vi "COM Error Checker.vi"(2 "error in (no error)":errorcluster, 3 "String In":string) -> (0 "error out":errorcluster, 1 "String":string)   [LabVIEW 2019, in "Instrument.KH7008.lvclass"]
uses:
  Instrument.KH7008.lvclass
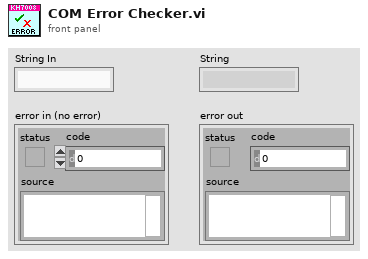
[diagram p1: front panel]
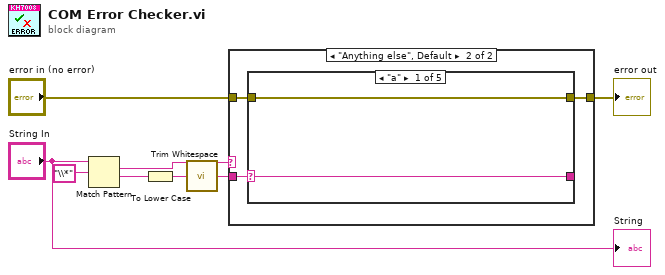
[diagram p0: block diagram]
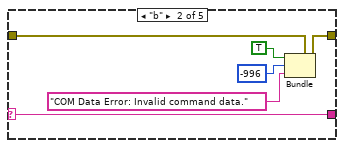
[diagram p3: hidden frame]
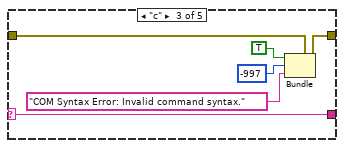
[diagram p4: hidden frame]
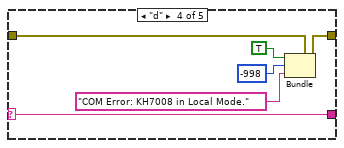
[diagram p5: hidden frame]
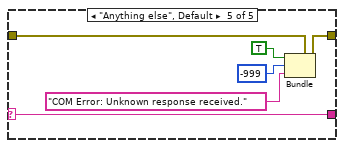
[diagram p6: hidden frame]
diagram:
  n1 = Match Pattern(string="String In", regular expression="\\*") -> (match substring=w2:string, after substring=w4:string)  [unwired: 1 in, 2 out]
  n2 = To Lower Case(string=w4) -> (all lower case string=w5:string)
  n3 = call <vilib>:"Trim Whitespace.vi"("string"=w5) -> ("trimmed string"=w6:string)  [unwired: 1 in]
  n4 = case shown="\"Anything else\", Default" w2 {
    tunnel: [w9 w12] -> w8
    tunnel: "error in (no error)" -> [w9 w11]
    tunnel: w6 -> [_ w10]
    frame "" {
    }
    frame "Anything else", Default {
      n5 = case shown="\"a\"" w10 {
        selector: w10 -> [w13 w16 w22 w28 w34]
        tunnel: w11 -> [w14 w20 w26 w32 w35]
        tunnel: [w14 w15 w21 w27 w33] -> w12
        tunnel: [w13 w16 w22 w28 w34] -> _
        frame "a" {
        }
        frame "b" {
          n6 = Bundle(cluster=w20, "status"=TRUE, "code"=-996, "source"="COM Data Error: Invalid command data.") -> (w15:errorcluster)
        }
        frame "c" {
          n7 = Bundle(cluster=w26, "status"=TRUE, "code"=-997, "source"="COM Syntax Error: Invalid command syntax.") -> (w21:errorcluster)
        }
        frame "d" {
          n8 = Bundle(cluster=w32, "status"=TRUE, "code"=-998, "source"="COM Error: KH7008 in Local Mode.") -> (w27:errorcluster)
        }
        frame "Anything else", Default {
          n9 = Bundle(cluster=w35, "status"=TRUE, "code"=-999, "source"="COM Error: Unknown response received.") -> (w33:errorcluster)
        }
      }
    }
  }
  "error out" <- w8
  "String" <- "String In"
